vi "ScopeStatus.vi"(8 "error in (no error)":errorcluster caption="错误输入（无错误）", 11 "handle":u64) -> (0 "error out":errorcluster caption="错误输出", 1 "ANIStatus":T1(ring), 2 "function return":i32, 3 "handle out":u64)   [LabVIEW 2018]
doc: "This function can get current scope's status. statedone means the data is ready"
uses:
  InstrumentsPlayground.lvlib
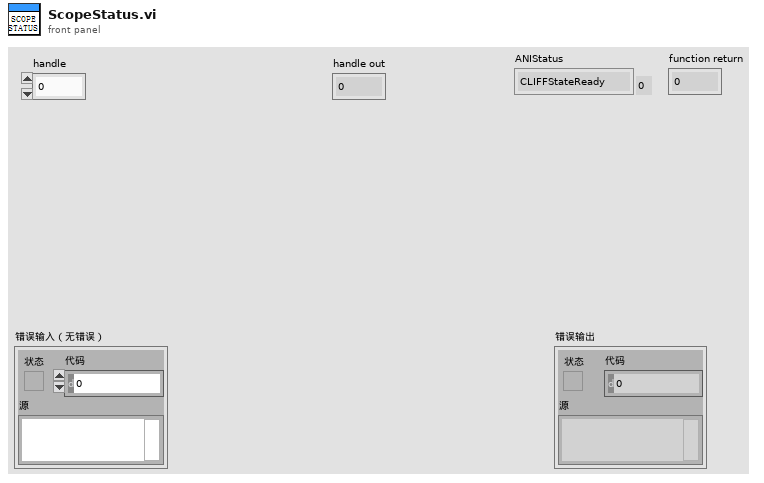
[diagram p1: front panel]
types:
  T1 = enum16{"CLIFFStateReady", "CLIFFStateArmed", "CLIFFStateDone", "CLIFFStateRunning", "CLIFFStateConfig", "CLIFFStatePrefill", "CLIFFStateTriggered", "CLIFFStateWait"}
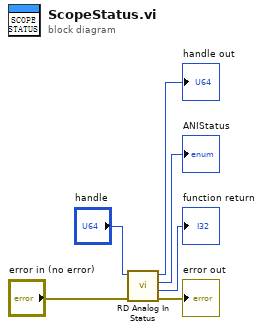
[diagram p0: block diagram]
diagram:
  n1 = call "RD Analog In Status.vi"("error in (no error)"="error in (no error)", "handle"="handle") -> ("error out"=→"error out":errorcluster, "function return"=→"function return":i32, "ANIStatus"=→"ANIStatus":T1, "handle out"=→"handle out":u64)  [unwired: 6 in]
